vi "Machining beam pointing camera-CK(StateMachine).vi"() -> ()   [LabVIEW 2009]
uses:
  <vilib>/userDefined/High Color/IMAQdx.ctl
  <vilib>/vision/Image Controls.llb/IMAQ Image.ctl
  <vilib>/Utility/error.llb/DialogType.ctl
  <vilib>/vision/driver/IMAQdx.llb/IMAQdx Buffer Number Mode.ctl
  <vilib>/vision/driver/IMAQdx.llb/IMAQdx Camera Control Mode.ctl
  <vilib>/vision/driver/IMAQdx.llb/IMAQdx Acquisition Mode.ctl
  <vilib>/vision/NI_Vision_Development_Module.lvlib
  <vilib>/vision/driver/NI_Vision_Acquisition_Software.lvlib
  Program Files/National Instruments/LabVIEW 2009/resource/objmgr/imaqdx.rc
panel:
  out "Global Report":T1 {"Mean Value" format="%.2f"; "%" format="%.2f"; "Area (calibrated)" format="%.2f"; "Maximal Value" format="%.2f"; "Minimal Value" format="%.2f"; "Standard Variation" format="%.2f"}
  out "Intensity Graph":i16[][](graph)
  out "Buffer Number Out":u32
  out "Camera Image":T2
  in  "Tab Control":T3(tab)=enum."Aquisition"
  in  "Include DS-string\nin filename":bool
  in  "Save Images":bool
  in  "Use\nGaussian <-> Centroid":bool
  in  "Set dev Limit\nto half Spotsize":bool
  out "Laser deviation":bool
  in  "Y dev limit":dbl=20.0
  in  "X dev limit":dbl=20.0
  out "Fast Buffer Means\nGaussian Fit":T4
  in  "Fast Buffer":i32=20
  out "Fit successful":bool
  out "XY Graph":cluster{i32[], "Best Gaussian Fit":dbl[]}[](graph)
  in  "Cursor 0 and Reference":u16(ring) items=["Do nothing", "Set Cursor 0 to Reference", "Set Reference to Cursor 0", "Set Reference and Cursor 0 to actual Position"]
  in  "Pause":bool
  out "Waveform Chart":i16(graph)
  out "X centroid pos":i32
  out "Y centroid pos":i32
  out "reference X index":dbl
  out "reference Y index":dbl
  in  "Activate Autoshutter":bool
  out "Shutter Value":dbl
  in  "OK":bool
  in  "Save One Image":bool
  out "Image":T2(plugin-control)
  out "Maximal Value":sgl
  in  "X parameter bounds":T5={"amp min"=0.0, "amp max"=inf, "center min"=0.0, "center max"=1288.0, "deviation min"=0.0, "deviation max"=300.0, "offset min"=0.0, "offset max"=inf}
  in  "Y parameter bounds":T5={"amp min"=0.0, "amp max"=inf, "center min"=0.0, "center max"=964.0, "deviation min"=0.0, "deviation max"=300.0, "offset min"=0.0, "offset max"=inf}
  in  "Slow Buffer":i32=1000
  out "Failed Fits":i32
  in  "Range":cluster{"Lower value":sgl, "Upper value":sgl}={"Lower value"=128.0, "Upper value"=255.0} {"Upper value" format="%.2f"; "Lower value" format="%.2f"}
  out "Centroid":cluster{"X Centroid":sgl, "Y Centroid":sgl} {"Y Centroid" format="%.2f"; "X Centroid" format="%.2f"}
  out "Slow Buffer\n Deviations":T4
  in  "Filename":string
  in  "Autoshutter Steps":enum32{"Relative", "Absolute"}(tab)=enum."Absolute"
  in  "%":dbl=10.0
  in  "ms":dbl=100.0
  in  "Image Buffer":u32=10
  in  "Device":T6="cam1"
  in  "Autoshutter Limits":cluster{"Upper Limit":i32, "Lopwer Limit":i32}={"Upper Limit"=3500, "Lopwer Limit"=1500}
  in  "Path":path=path "C:/Temp/ImagesCK"
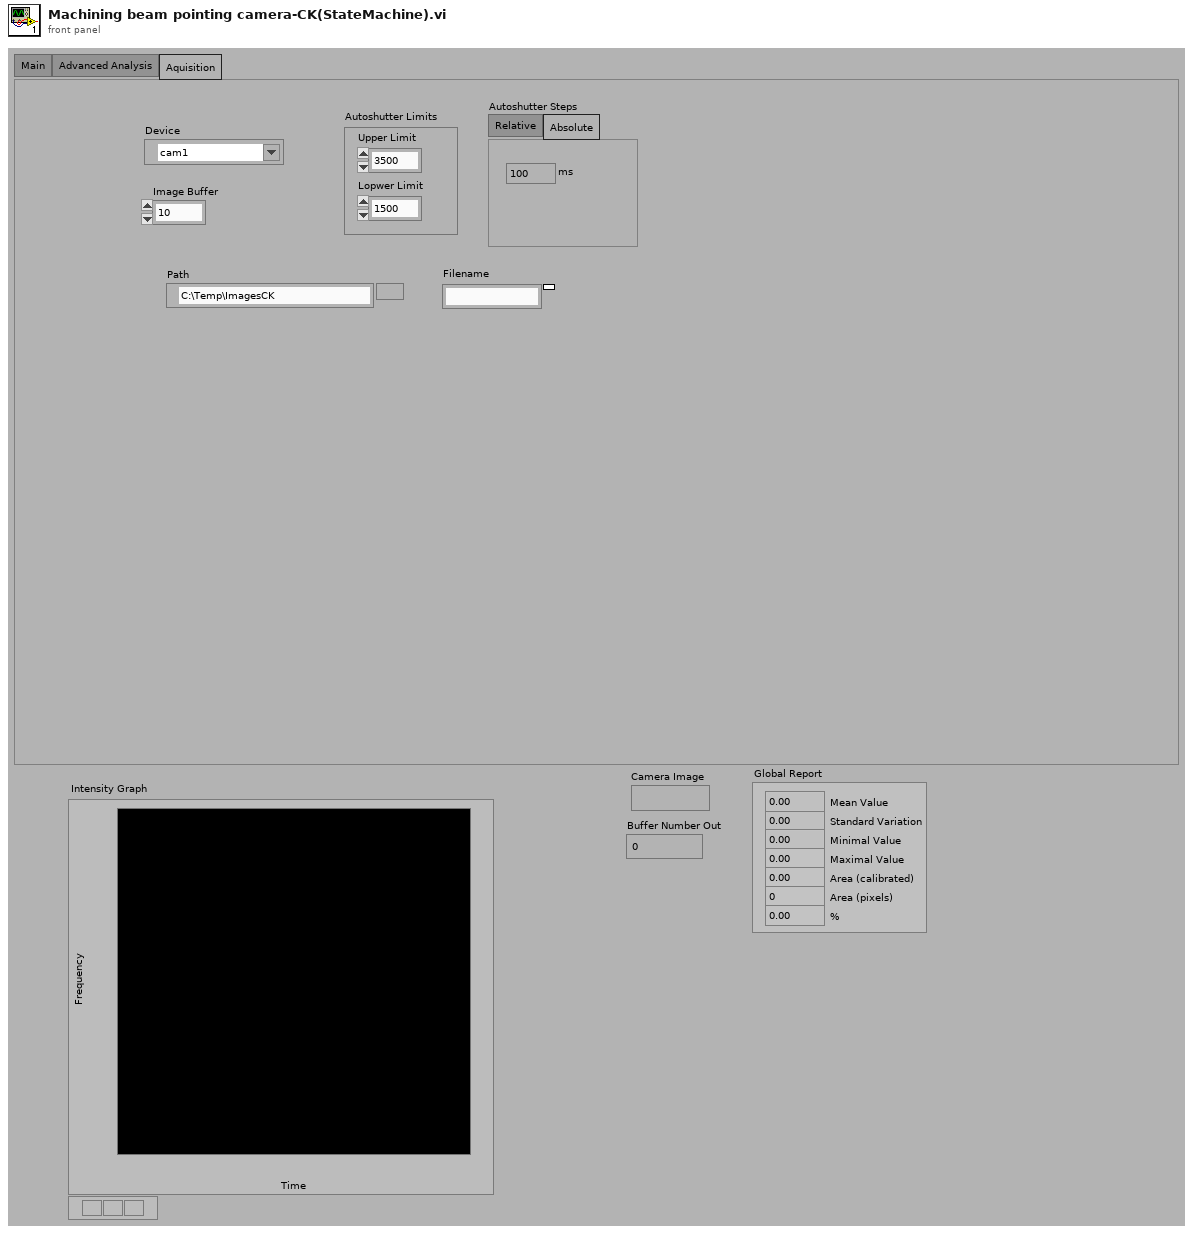
[diagram p1: front panel]
types:
  T1 = cluster{"Mean Value":sgl, "Standard Variation":sgl, "Minimal Value":sgl, "Maximal Value":sgl, "Area (calibrated)":sgl, "Area (pixels)":i32, "%":sgl}
  T2 = typedef "IMAQ Image.ctl" = refnum<image>
  T3 = enum32{"Main", "Advanced Analysis", "Aquisition"}
  T4 = cluster{"Y-AMplitude":dbl, "Y-deviation":dbl, "Y-position":dbl, "X-Amplitude":dbl, "X-deviation":dbl, "X-Position":dbl}
  T5 = cluster{"amp min":dbl, "amp max":dbl, "center min":dbl, "center max":dbl, "deviation min":dbl, "deviation max":dbl, "offset min":dbl, "offset max":dbl}
  T6 = typedef "IMAQdx.ctl" = refnum<k21>
  T7 = enum32{"invalid app kind", "Development System", "Run Time System", "Student Edition", "Embedded LabVIEW", "Evaluation", "Custom"}
  T8 = enum32{"Invalid", "Standard", "Closed", "Hidden", "Minimized", "Maximized"}
  T9 = typedef "NI_Vision_Acquisition_Software.lvlib/IMAQdx Buffer Number Mode.ctl" = enum32{"Next", "Last", "Buffer Number"}
  T10 = typedef "NI_Vision_Acquisition_Software.lvlib/IMAQdx Camera Control Mode.ctl" = enum32{"Controller", "Listener"}
  T11 = typedef "NI_Vision_Acquisition_Software.lvlib/IMAQdx Acquisition Mode.ctl" = enum32{"One Shot", "Continuous"}
  T12 = cluster{"Core":cluster{"Current VI Reference":refnum<vi>, "Close Panel on Exit?":bool}, "IMAQdx Session":T6, "Camera Image":T2, "Threshold Image":T2, "Framecount":u64, "Gaussian Result":cluster{cluster{"Y-amplitude":dbl, "Y-standard deviation":dbl, "Y-center":dbl}, cluster{"X-amplitude":dbl, "X-standard deviation":dbl, "X-center":dbl}}, "Global Report":cluster{"Mean Value":sgl, "Standard Variation":sgl, "Minimal Value":sgl, "Maximal Value":sgl, "Area (calibrated)":sgl, "Area (pixels)":i32, "%":sgl}, "Centroid":cluster{"X Centroid":sgl, "Y Centroid":sgl}, "DataBuffer":cluster{cluster{"Y-amplitude":dbl, "Y-standard deviation":dbl, "Y-center":dbl}, cluster{"X-amplitude":dbl, "X-standard deviation":dbl, "X-center":dbl}}[], "Fast Buffer Results":cluster{"Y-AMplitude":dbl, "Y-deviation":dbl, "Y-position":dbl, "X-Amplitude":dbl, "X-deviation":dbl, "X-Position":dbl}}
  T13 = typedef "DialogType.ctl" = u16
  T14 = cluster{cluster{"Y-amplitude":dbl, "Y-standard deviation":dbl, "Y-center":dbl}, cluster{"X-amplitude":dbl, "X-standard deviation":dbl, "X-center":dbl}}
  T15 = cluster{cluster{"Y-amplitude":dbl, "Y-standard deviation":dbl, "Y-center":dbl}, cluster{"X-amplitude":dbl, "X-standard deviation":dbl, "X-center":dbl}}[]
  T16 = cluster{"Current VI Reference":refnum<vi>, "Close Panel on Exit?":bool}
  T17 = cluster{"reference X index ":dbl, "reference Y index ":dbl}
  T18 = typedef "LVPointDoubleTypeDef.ctl" = cluster{"Cursor X":dbl, "Cursor Y":dbl}
  T19 = cluster{"X centroid pos":i32, "Y centroid pos":i32}
  T20 = typedef "Image Type" = u32
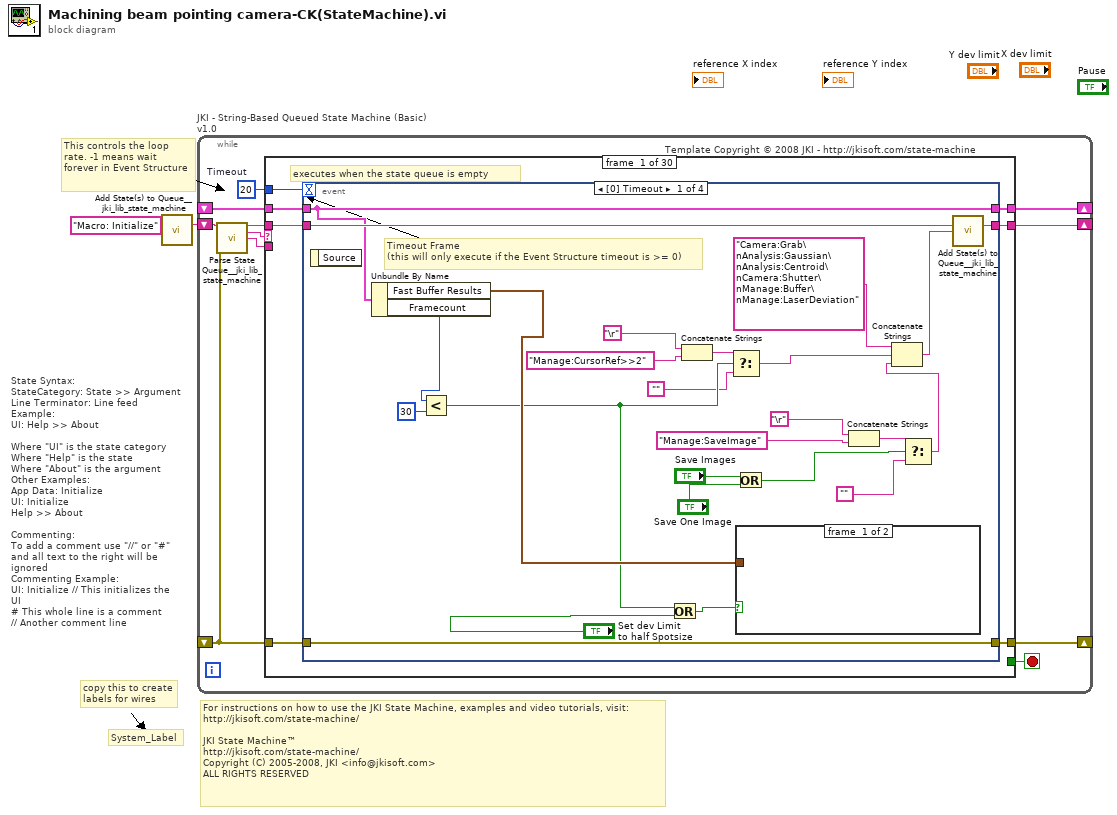
[diagram p0: block diagram]
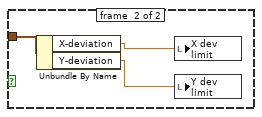
[diagram p2: hidden frame]
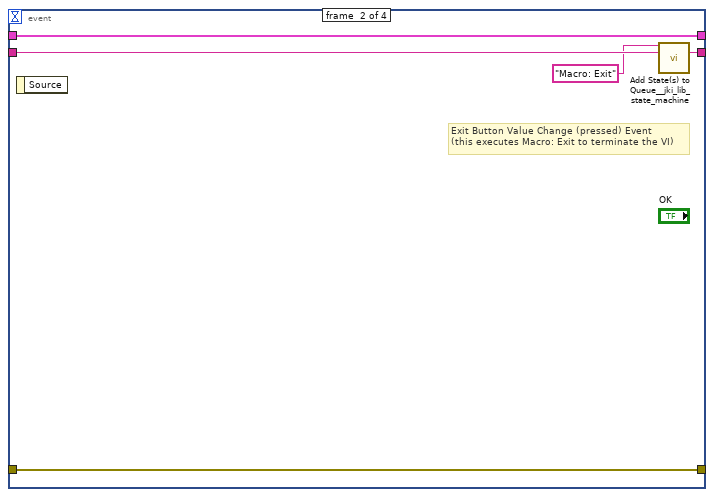
[diagram p3: hidden frame]
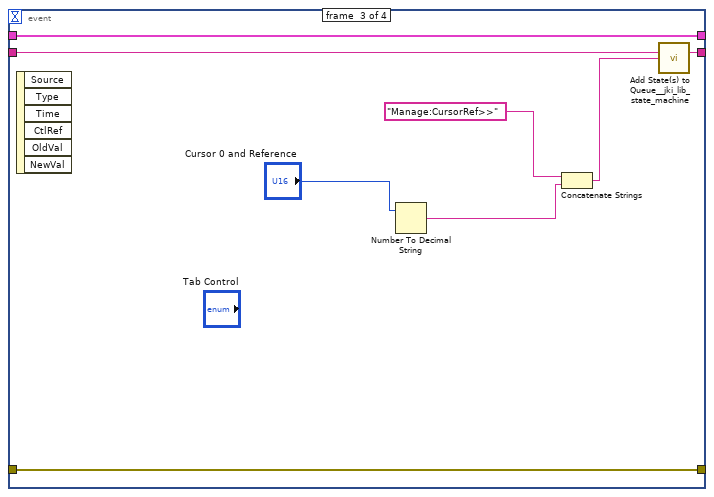
[diagram p4: hidden frame]
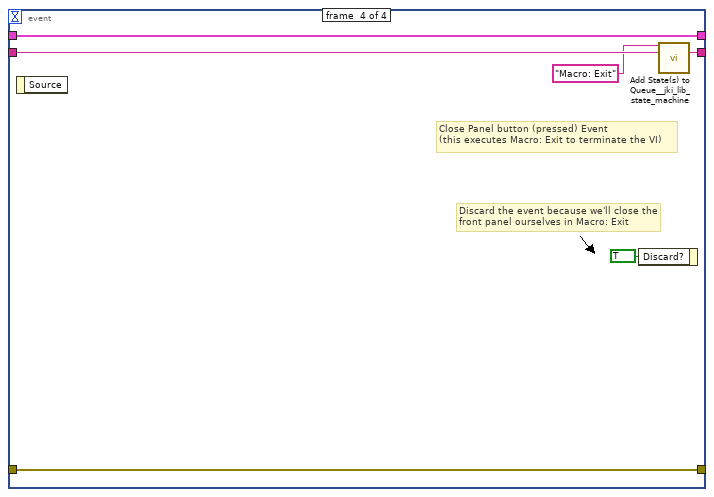
[diagram p5: hidden frame]
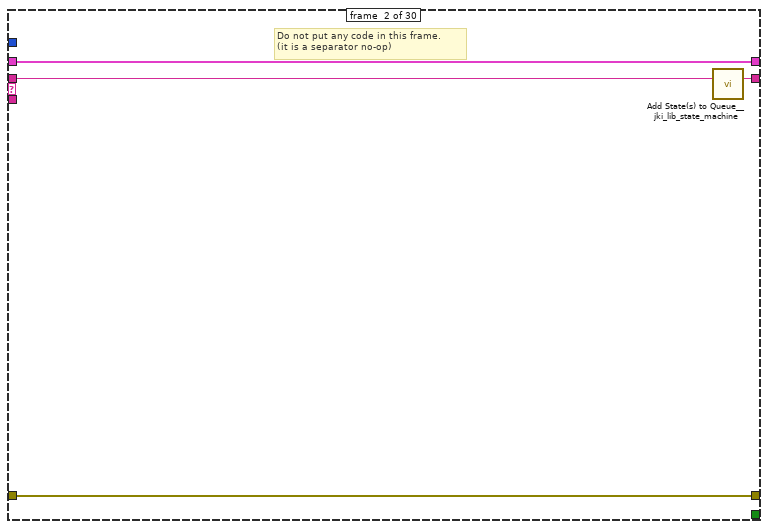
[diagram p6: hidden frame]
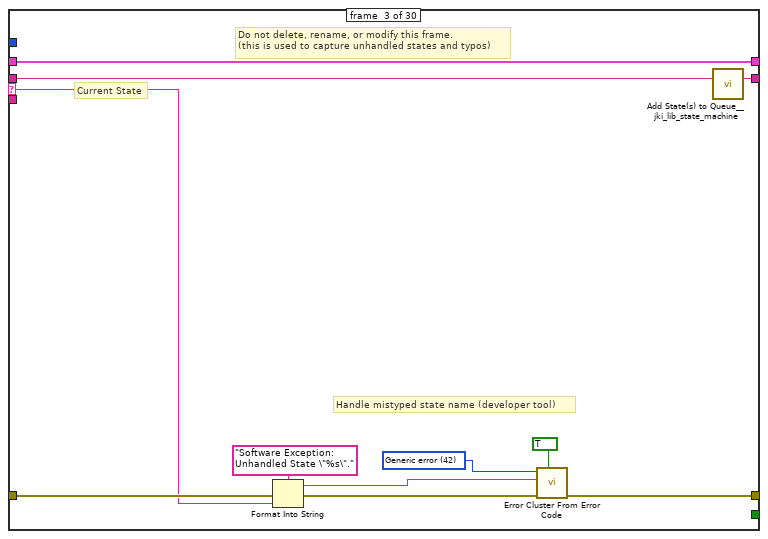
[diagram p7: hidden frame]
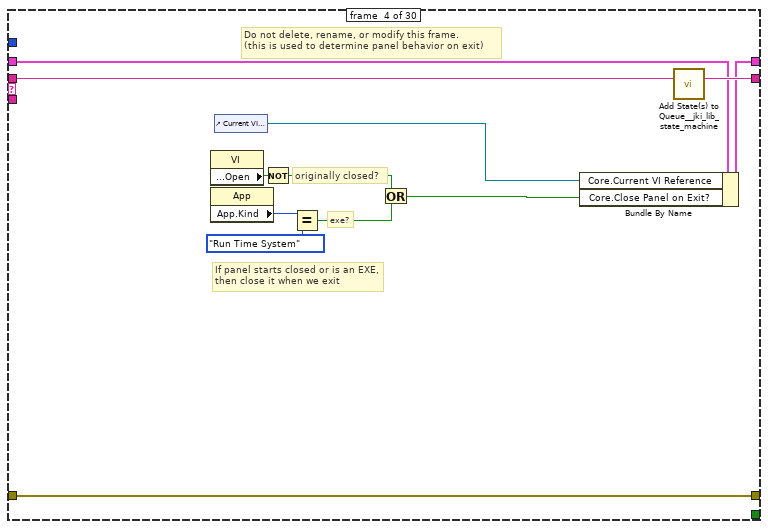
[diagram p8: hidden frame]
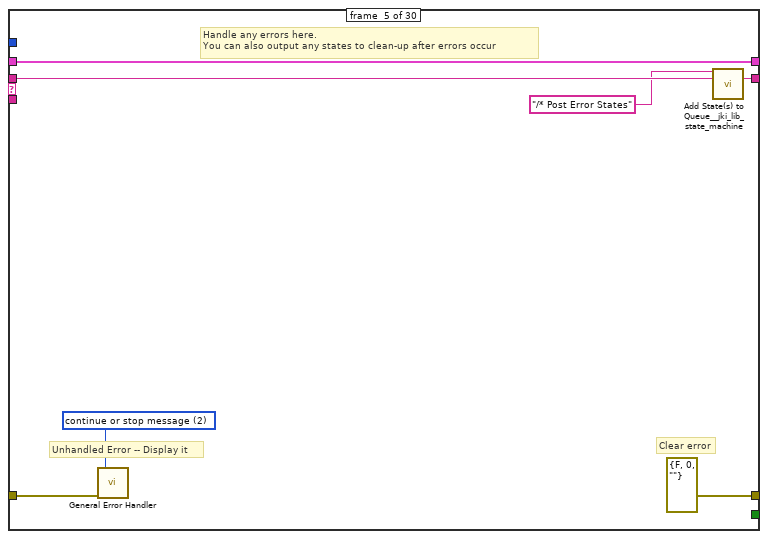
[diagram p9: hidden frame]
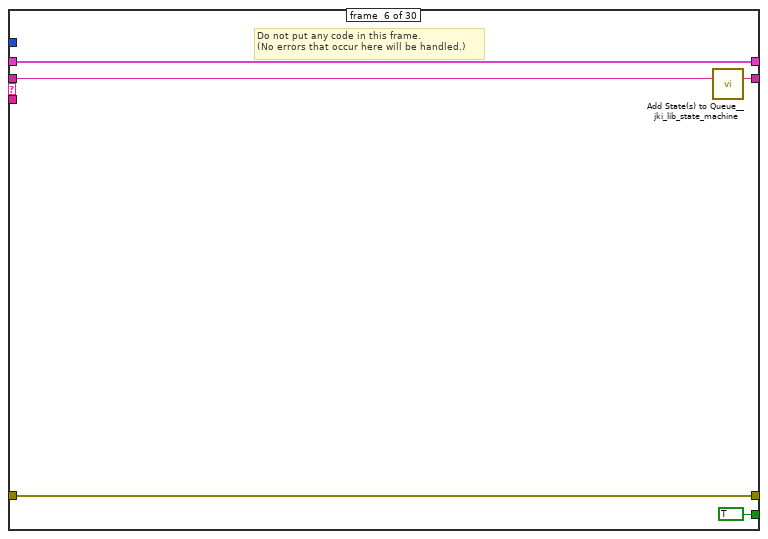
[diagram p10: hidden frame]
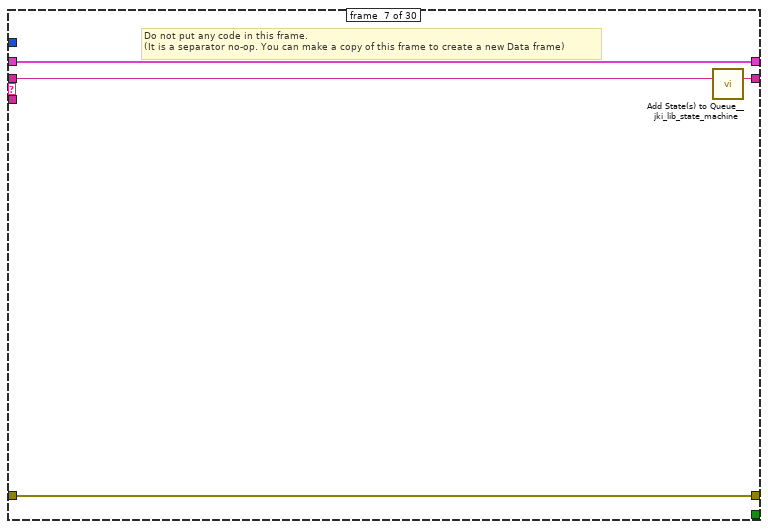
[diagram p11: hidden frame]
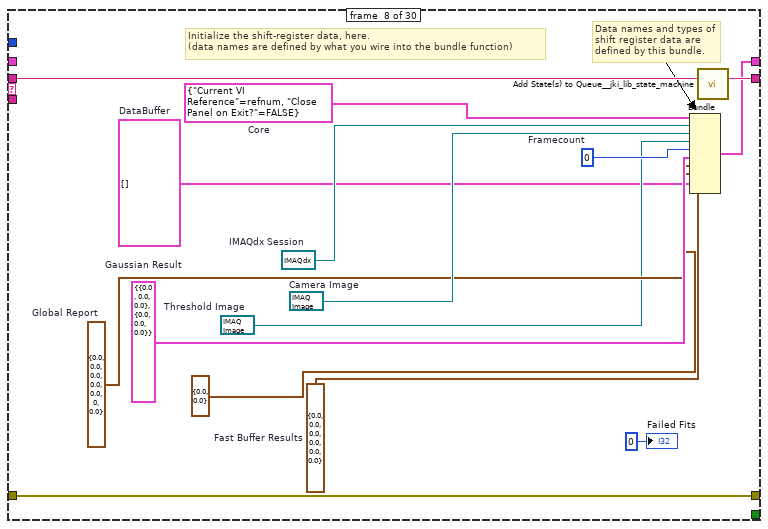
[diagram p12: hidden frame]
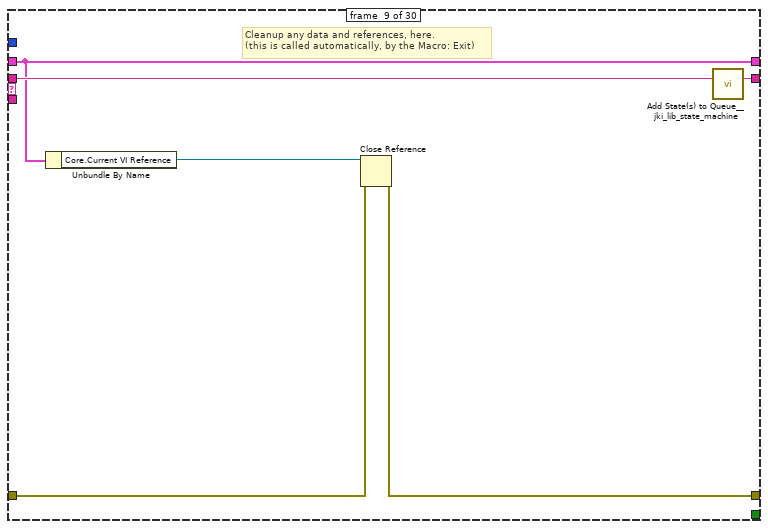
[diagram p13: hidden frame]
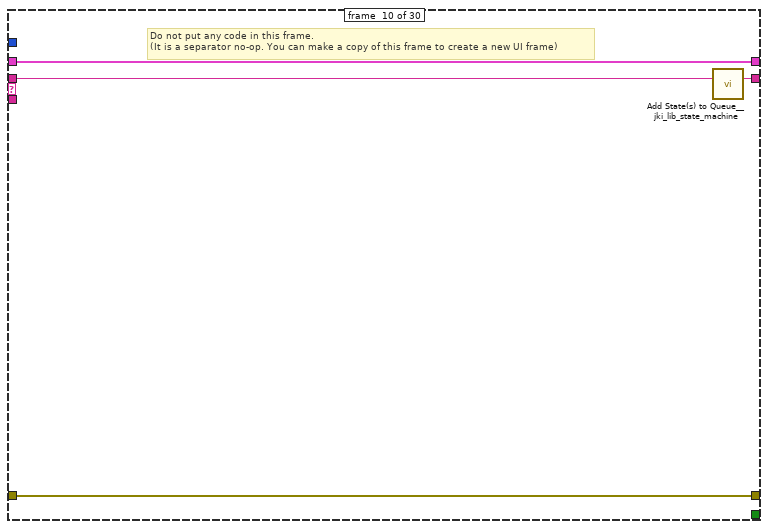
[diagram p14: hidden frame]
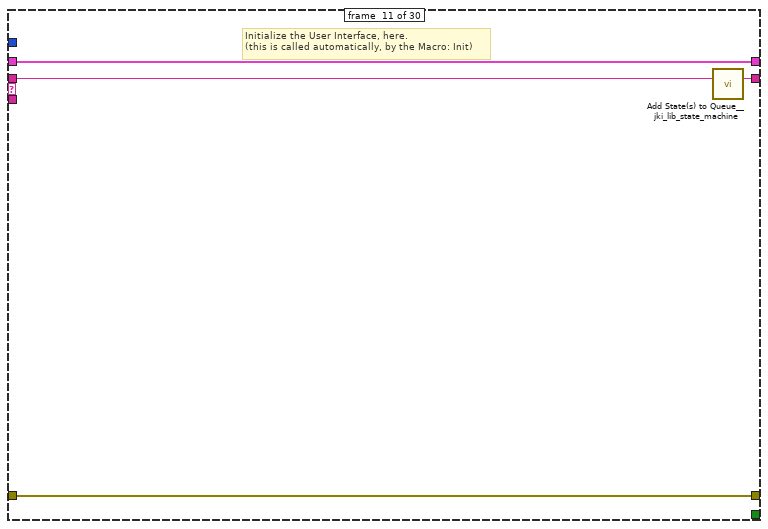
[diagram p15: hidden frame]
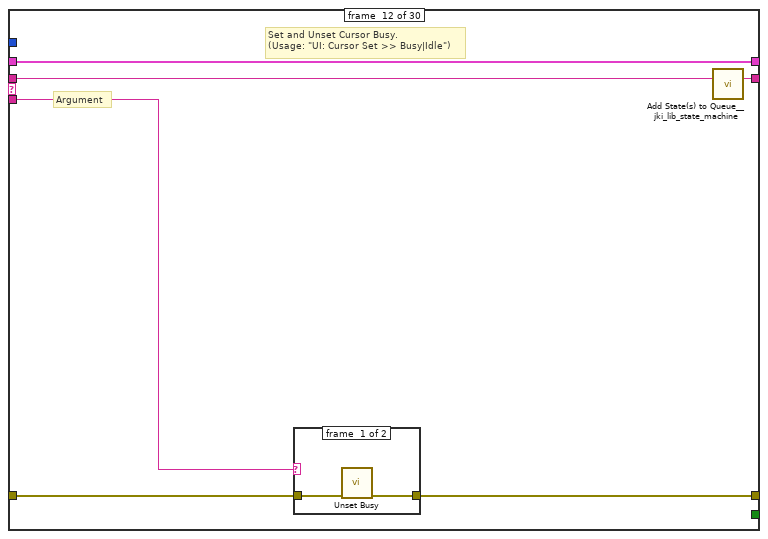
[diagram p16: hidden frame]
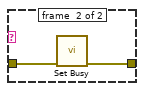
[diagram p17: hidden frame]
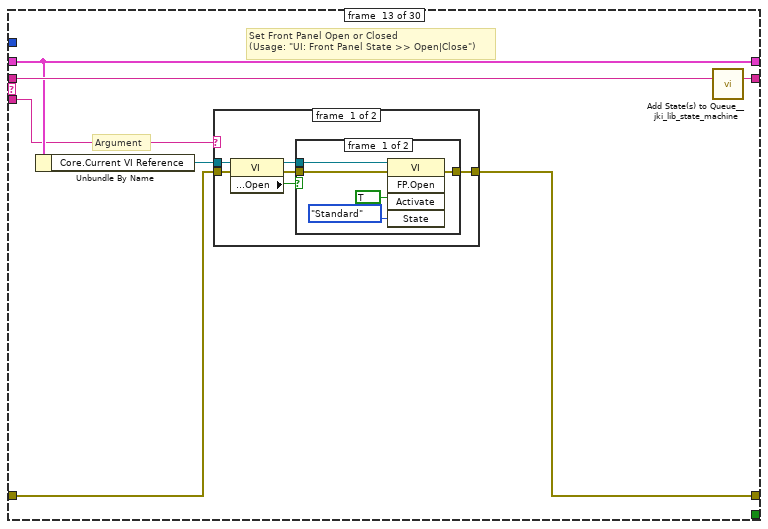
[diagram p18: hidden frame]
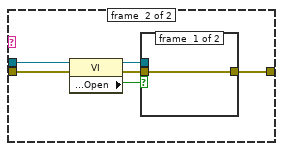
[diagram p20: hidden frame]
diagram:
  # "For instructions on how to use the JKI State Machine, examples and video tutorials, visit:\nhttp://jkisoft.com/state-machine/\n\nJKI State Machine™\nhttp://jkisoft.com/state-machine/\nCopyright (C) 2005-2008, JKI <info@jkisoft.com>\nALL RIGHTS RESERVED"
  # "State Syntax:\nStateCategory: State >> Argument\nLine Terminator: Line feed\nExample:\nUI: Help >> About\n\nWhere \"UI\" is the state category\nWhere \"Help\" is the state\nWhere \"About\" is the argument\nOther Examples:\nApp Data: Initialize\nUI: Initialize\nHelp >> About\n\nCommenting:\nTo add a comment use \"//\" or \"#\" and all text to the right will be ignored\nCommenting Example:\nUI: Initialize // This initializes the UI\n# This whole line is a comment\n// Another comment line"
  # "copy this to create labels for wires"
  # "This controls the loop rate. -1 means wait forever in Event Structure"
  # "System_Label"
  n1 = call <vilib>:"Add State(s) to Queue__jki_lib_state_machine.vi"("State(s) in (\"\")"="Macro: Initialize") -> ("States Out"=w2:string)  [unwired: 14 in]
  n2 = while "JKI - String-Based Queued State Machine (Basic) v1.0" {
    shift-right: [w6] -> _
    shift-left: _ -> [w5]
    shift-right: [w9] -> _
    shift-left: _ -> [w3]
    shift-right: [w8] -> _
    shift-left: w2 -> [w10]
    stop <- w7 stop-if-true
    w4 = 20  # Timeout
    # "Template Copyright © 2008 JKI - http://jkisoft.com/state-machine"
    n3 = call <vilib>:"Parse State Queue__jki_lib_state_machine.vi"("State Queue"=w10, "Error In (no error)"=w3) -> ("Remaining States"=w12:string, "Current State"=w13:string, "Arguments"=w11:string)  [unwired: 11 in]
    n4 = case shown="\"Analysis:Centroid\"" w13 {
      selector: w13 -> [_ _ w72 _ _ _ _ _ _ _ _ _ _ _ _ _ _ _ _ _ _ _ _ _ _ _ _ _ _ _]
      tunnel: w12 -> [w20 w71 w76 w94 w101 w106 w110 w125 w131 w135 w139 w145 w156 w182 w187 w197 w201 w236 w259 w294 w326 w330 w348 w359 w365 w369 w387 w406 w441 w452]
      tunnel: w11 -> [_ _ _ _ _ _ _ _ _ _ _ w140 w150 _ _ _ _ _ w253 _ _ _ _ _ _ _ _ _ _ _]
      tunnel: w5 -> [w18 w68 w74 w85 w98 w104 w107 _ w126 w132 w137 w143 w152 w179 w184 w194 w198 w231 w255 w282 w323 w327 w346 w356 w362 w366 w385 w404 w439 w445]
      tunnel: [w17 w69 w78 w91 errorcluster {"status"=FALSE, "code"=0, "source"=""} ("error out") w103 w108 w118 w127 w133 w136 w141 w153 w180 w185 w195 w199 w233 w256 w283 w324 w328 w333 w357 w363 w367 w375 w391 w420 w446] -> w9
      tunnel: w3 -> [w16 w69 w77 w91 w97 w103 w108 w118 w128 w133 w136 w142 w154 w180 w185 w195 w199 w222 w257 w284 w324 w328 w341 w357 w363 w367 w380 w392 w427 w444]
      tunnel: [w19 w70 w75 w93 w100 w105 w109 w124 w130 w134 w138 w144 w155 w181 w186 w196 w200 w235 w258 w293 w325 w329 w347 w358 w364 w368 w386 w405 w440 w451] -> w8
      tunnel: [_ _ _ _ _ TRUE _ _ _ _ _ _ _ _ _ _ _ _ _ _ _ _ _ _ _ _ _ _ _ _] -> w7
      tunnel: [w15 w68 w74 w92 w98 w104 w107 w123 w126 w132 w137 w143 w152 w179 w184 w194 w198 w230 w255 w282 w322 w327 w345 w355 w362 w366 w384 w403 w438 w445] -> w6
      tunnel: w4 -> [w14 _ _ _ _ _ _ _ _ _ _ _ _ _ _ _ _ _ _ _ _ _ _ _ _ _ _ _ _ _]
      frame #0 {
        # "executes when the state queue is empty"
        n5 = event shown="[0] Timeout" {
          selector: _ -> [_ _ _ _]
          dyn-events: _ -> [_ _ _ _]
          timeout: w14 -> [_ _ _ _]
          tunnel: w20 -> [w45 w53 w61 w67]
          tunnel: [w44 w52 w60 w66] -> w19
          tunnel: w18 -> [w37 w50 w58 w64]
          tunnel: [w43 w51 w59 w65] -> w17
          tunnel: w16 -> [w43 w51 w59 w65]
          tunnel: [w37 w50 w58 w64] -> w15
          event #0 {
            # "Timeout Frame\n(this will only execute if the Event Structure timeout is >= 0)"
            n6 = event-data() -> ()  [unwired: 1 in, 1 out]
            n7 = Unbundle By Name(w37) -> ("Fast Buffer Results"=w40:T4, "Framecount"=w38:u64)
            n8 = Less?(x=w38, y=u64 30) -> (x < y?=w35:bool)
            n9 = Or(x=w35, y="Set dev Limit\nto half Spotsize") -> (x .or. y?=w41:bool)
            n10 = Concatenate Strings("\r", "Manage:CursorRef>>2" ("State(s) at Back (\"\")")) -> (w31:string)
            n11 = Select(t=w31, s=w35, f="") -> (s? t:f=w30:string)
            n12 = Or(x="Save Images", y="Save One Image") -> (x .or. y?=w21:bool)
            n13 = case shown="True" w41 {
              tunnel: w40 -> [_ w46]
              frame #0 {
              }
              frame #1 {
                n14 = Unbundle By Name(w46) -> ("X-deviation"=w47:dbl, "Y-deviation"=w48:dbl)
                n15 = local write "X dev limit"(w47) -> ()
                n16 = local write "Y dev limit"(w48) -> ()
              }
            }
            n17 = Concatenate Strings("\r", "Manage:SaveImage" ("State(s) at Back (\"\")")) -> (w28:string)
            n18 = Select(t=w28, s=w21, f="") -> (s? t:f=w24:string)
            n19 = Concatenate Strings("Camera:Grab\nAnalysis:Gaussian\nAnalysis:Centroid\nCamera:Shutter\nManage:Buffer\nManage:LaserDeviation" ("State(s) at Back (\"\")"), w30, w24) -> (w29:string)
            n20 = call <vilib>:"Add State(s) to Queue__jki_lib_state_machine.vi"("State(s) in (\"\")"=w45, "State(s) at Back (\"\")"=w29) -> ("States Out"=w44:string)  [unwired: 13 in]
          }
          event #1 {
            # "Exit Button Value Change (pressed) Event\n(this executes Macro: Exit to terminate the VI)"
            n21 = event-data() -> ()  [unwired: 1 in, 1 out]
            n22 = call <vilib>:"Add State(s) to Queue__jki_lib_state_machine.vi"("State(s) in Front (\"\")"="Macro: Exit", "State(s) in (\"\")"=w53) -> ("States Out"=w52:string)  [unwired: 13 in]
          }
          event #2 {
            n23 = event-data() -> ()  [unwired: 1 in, 6 out]
            n24 = Number To Decimal String(number="Cursor 0 and Reference") -> (decimal integer string=w56:string)  [unwired: 1 in]
            n25 = Concatenate Strings("Manage:CursorRef>>" ("State(s) at Back (\"\")"), w56) -> (w54:string)
            n26 = call <vilib>:"Add State(s) to Queue__jki_lib_state_machine.vi"("State(s) in (\"\")"=w61, "State(s) at Back (\"\")"=w54) -> ("States Out"=w60:string)  [unwired: 13 in]
          }
          event #3 {
            # "Discard the event because we'll close the front panel ourselves in Macro: Exit"
            # "Close Panel button (pressed) Event\n(this executes Macro: Exit to terminate the VI)"
            n27 = event-data() -> ()  [unwired: 1 in, 1 out]
            n28 = event-data("Discard?"=TRUE) -> ()  [unwired: 1 in, 1 out]
            n29 = call <vilib>:"Add State(s) to Queue__jki_lib_state_machine.vi"("State(s) in Front (\"\")"="Macro: Exit", "State(s) in (\"\")"=w67) -> ("States Out"=w66:string)  [unwired: 13 in]
          }
        }
      }
      frame #1 {
        # "Do not put any code in this frame.\n(it is a separator no-op)"
        n30 = call <vilib>:"Add State(s) to Queue__jki_lib_state_machine.vi"("State(s) in (\"\")"=w71) -> ("States Out"=w70:string)  [unwired: 14 in]
      }
      frame #2 {
        w81 = 42 items=["No error", "Argument error", "Memory is full", "Out of zone", "End of file", "File already open", "Generic file I/O error", "File not found", "File permission error", "Disk is full", "Duplicate path", "Too many files open", "System feature not enabled", "Resource file not found", "Cannot add resource", "Resource not found", "Image not found", "Image memory error", "Pen does not exist", "Config type invalid", "Config token not found", "Config parse error", "Config memory error", "Bad external code format", "Bad external code offset", "External code not present", "Null window", "Destroy window error", "Null menu", "Print aborted", "Bad print record", "Print driver error", "Windows error during printing", "Memory error during printing", "Print dialog error", "Generic print error", "Invalid device refnum", "Device not found", "Device parameter error", "Device unit error", "Cannot open device", "Device call aborted", "Generic error", "Cancelled by user", "Object ID too low", "Object ID too high", "Object not in heap", "Unknown heap", "Unknown object (invalid DefProc)", "Unknown object (DefProc not in table)", "Message out of range", "Invalid (null) method", "Unknown message", "Manager call not supported", "Bad address", "Network operation in progress", "Network operation timed out", "Connection is busy", "Network attribute not supported", "Network error", "Address in use", "System out of memory", "Connection aborted", "Connection refused", "Not connected", "Already connected", "Connection closed", "Initialization error (interapplication manager)", "Bad occurrence", "Wait on unbound occurrence handler", "Occurrence queue overflow", "Datalog type conflict", "Unused", "Unrecognized type (interapplication manager)", "Memory corrupt", "Failed to make temporary DLL", "Old CIN version", "Drag socket not found", "Failed to load drop-object", "Failed to register OLE object", "Failed to release OLE object", "Format specifier type mismatch", "Unknown format specifier", "Too few format specifiers", "Too many format specifiers", "Scan failed", "Newer CIN version", "Error converting to variant", "Runtime menu error", "Password tampered", "Variant attribute not found", "Incompatible variant data type", "Event data is not available", "Event Store is not present", "Occurrence is not found", "Event Queue is not created", "Event info is not available", "Refnum passed is NULL", "Error retrieving Class GUID", "Error retrieving CoClass GUID", "Error retrieving TypeLib GUID.", "Bad built application magic bytes.", "Specific driver is different from the specific driver associated with the Logical Name.", "There is no session opened to the class driver.", "Max Error", "MAX - Error with config objects", "MAX - Error loading configuration", "MAX - Group not supported"]
        # "Current State"
        # "Do not delete, rename, or modify this frame.\n(this is used to capture unhandled states and typos)"
        # "Handle mistyped state name (developer tool)"
        n31 = Format Into String(format string="Software Exception: Unhandled State \"%s\"." ("message"), error in=w77, w72) -> (resulting string=w80:string, error out=w79:errorcluster)  [unwired: 1 in]
        n32 = call <vilib>:"Error Cluster From Error Code.vi"("show call chain? (False)"=TRUE, "error in (no error)"=w79, "error message (\"\")"=w80, "error code (0)"=w81) -> ("error out"=w78:errorcluster)  [unwired: 5 in]
        n33 = call <vilib>:"Add State(s) to Queue__jki_lib_state_machine.vi"("State(s) in (\"\")"=w76) -> ("States Out"=w75:string)  [unwired: 14 in]
      }
      frame #3 {
        # "Do not delete, rename, or modify this frame.\n(this is used to determine panel behavior on exit)"
        # "originally closed?"
        # "exe?"
        # "If panel starts closed or is an EXE, then close it when we exit"
        n34 = property class="VI"() -> ("Front Panel.Open"=w90:bool)  [unwired: 2 in, 2 out]
        n35 = property class="App"() -> ("App.Kind"=w89:T7)  [unwired: 2 in, 2 out]
        n36 = control-ref of="Current VI Reference"() -> (w83:refnum<vi>)
        n37 = Not(x=w90) -> (.not. x?=w87:bool)
        n38 = Equal?(x=w89, y=T7."Run Time System" ("Application:Kind")) -> (x = y?=w86:bool)
        n39 = Or(x=w87, y=w86) -> (x .or. y?=w84:bool)
        n40 = Bundle By Name(cluster=w85, "Core.Current VI Reference"=w83, "Core.Close Panel on Exit?"=w84) -> (w92:T12)
        n41 = call <vilib>:"Add State(s) to Queue__jki_lib_state_machine.vi"("State(s) in (\"\")"=w94) -> ("States Out"=w93:string)  [unwired: 14 in]
      }
      frame #4 {
        w95 = T13 2 items=["no dialog", "OK message", "continue or stop message", "OK message + warnings", "continue/stop + warnings"] ("type of dialog (OK msg:1)")
        # "Unhandled Error -- Display it"
        # "Handle any errors here.\nYou can also output any states to clean-up after errors occur"
        # "Clear error"
        n42 = call <vilib>:"General Error Handler.vi"("type of dialog (OK msg:1)"=w95, "error in (no error)"=w97) -> ()  [unwired: 9 in, 5 out]
        n43 = call <vilib>:"Add State(s) to Queue__jki_lib_state_machine.vi"("State(s) in Front (\"\")"="/* Post Error States", "State(s) in (\"\")"=w101) -> ("States Out"=w100:string)  [unwired: 13 in]
      }
      frame #5 {
        # "Do not put any code in this frame.\n(No errors that occur here will be handled.)"
        n44 = call <vilib>:"Add State(s) to Queue__jki_lib_state_machine.vi"("State(s) in (\"\")"=w106) -> ("States Out"=w105:string)  [unwired: 14 in]
      }
      frame #6 {
        # "Do not put any code in this frame.\n(It is a separator no-op. You can make a copy of this frame to create a new Data frame)"
        n45 = call <vilib>:"Add State(s) to Queue__jki_lib_state_machine.vi"("State(s) in (\"\")"=w110) -> ("States Out"=w109:string)  [unwired: 14 in]
      }
      frame #7 {
        w112 = T4 {"Y-AMplitude"=0.0, "Y-deviation"=0.0, "Y-position"=0.0, "X-Amplitude"=0.0, "X-deviation"=0.0, "X-Position"=0.0}  # Fast Buffer Results
        w114 = T2 refnum  # Threshold Image
        w116 = T1 {"Mean Value"=0.0, "Standard Variation"=0.0, "Minimal Value"=0.0, "Maximal Value"=0.0, "Area (calibrated)"=0.0, "Area (pixels)"=0, "%"=0.0}  # Global Report
        w117 = T14 {{"Y-amplitude"=0.0, "Y-standard deviation"=0.0, "Y-center"=0.0}, {"X-amplitude"=0.0, "X-standard deviation"=0.0, "X-center"=0.0}}  # Gaussian Result
        w119 = T2 refnum  # Camera Image
        w120 = T6 refnum  # IMAQdx Session
        w121 = u64 0  # Framecount
        w113 = T15 []  # DataBuffer
        w122 = T16 {"Current VI Reference"=refnum, "Close Panel on Exit?"=FALSE}  # Core
        # "Data names and types of shift register data are defined by this bundle."
        # "Initialize the shift-register data, here.\n(data names are defined by what you wire into the bundle function)"
        n46 = Bundle("Core"=w122, "IMAQdx Session"=w120, "Camera Image"=w119, "Threshold Image"=w114, "Framecount"=w121, "Gaussian Result"=w117, "Global Report"=w116, "Centroid"=cluster{"X Centroid":sgl, "Y Centroid":sgl} {"X Centroid"=0.0, "Y Centroid"=0.0}, "DataBuffer"=w113, "Fast Buffer Results"=w112) -> (w123:T12)  [unwired: 1 in]
        n47 = call <vilib>:"Add State(s) to Queue__jki_lib_state_machine.vi"("State(s) in (\"\")"=w125) -> ("States Out"=w124:string)  [unwired: 14 in]
        "Failed Fits" <- 0 ("Failed Fits")
      }
      frame #8 {
        # "Cleanup any data and references, here.\n(this is called automatically, by the Macro: Exit)"
        n48 = Unbundle By Name(w126) -> ("Core.Current VI Reference"=w129:refnum<vi>)
        n49 = Close Reference(reference=w129, error in (no error)=w128) -> (error out=w127:errorcluster)
        n50 = call <vilib>:"Add State(s) to Queue__jki_lib_state_machine.vi"("State(s) in (\"\")"=w131) -> ("States Out"=w130:string)  [unwired: 14 in]
      }
      frame #9 {
        # "Do not put any code in this frame.\n(It is a separator no-op. You can make a copy of this frame to create a new UI frame)"
        n51 = call <vilib>:"Add State(s) to Queue__jki_lib_state_machine.vi"("State(s) in (\"\")"=w135) -> ("States Out"=w134:string)  [unwired: 14 in]
      }
      frame #10 {
        # "Initialize the User Interface, here.\n(this is called automatically, by the Macro: Init)"
        n52 = call <vilib>:"Add State(s) to Queue__jki_lib_state_machine.vi"("State(s) in (\"\")"=w139) -> ("States Out"=w138:string)  [unwired: 14 in]
      }
      frame #11 {
        # "Argument"
        # "Set and Unset Cursor Busy.\n(Usage: \"UI: Cursor Set >> Busy|Idle\")"
        n53 = case shown="\"Idle\", Default" w140 {
          tunnel: w142 -> [w147 w149]
          tunnel: [w146 w148] -> w141
          frame #0 {
            n54 = call <vilib>:"Unset Busy.vi"("error in (no error)"=w147) -> ("error out"=w146:errorcluster)  [unwired: 10 in]
          }
          frame #1 {
            n55 = call <vilib>:"Set Busy.vi"("error in (no error)"=w149) -> ("error out"=w148:errorcluster)  [unwired: 9 in, 1 out]
          }
        }
        n56 = call <vilib>:"Add State(s) to Queue__jki_lib_state_machine.vi"("State(s) in (\"\")"=w145) -> ("States Out"=w144:string)  [unwired: 14 in]
      }
      frame #12 {
        # "Argument"
        # "Set Front Panel Open or Closed\n(Usage: \"UI: Front Panel State >> Open|Close\")"
        n57 = Unbundle By Name(w152) -> ("Core.Current VI Reference"=w151:refnum<vi>)
        n58 = case shown="\"Open\", Default" w150 {
          tunnel: w154 -> [w160 w173]
          tunnel: [w162 w174] -> w153
          tunnel: w151 -> [w161 w171]
          frame #0 {
            n59 = property class="VI"(reference=w161, error in=w160) -> (reference out=w158:refnum<vi>, error out=w159:errorcluster, "Front Panel.Open"=w157:bool)
            n60 = case shown="False" w157 {
              tunnel: [w165 w168] -> w162
              tunnel: w159 -> [w164 w168]
              tunnel: w158 -> [w163 _]
              frame #0 {
                n61 = invoke class="VI" method="FP.Open"(reference=w163, error in=w164, "Activate"=TRUE, "State"=T8."Standard") -> (error out=w165:errorcluster)  [unwired: 1 in, 4 out]
              }
              frame #1 {
              }
            }
          }
          frame #1 {
            n62 = property class="VI"(reference=w171, error in=w173) -> (reference out=w170:refnum<vi>, error out=w172:errorcluster, "Front Panel.Open"=w169:bool)
            n63 = case shown="True" w169 {
              tunnel: [w175 w178] -> w174
              tunnel: w172 -> [w175 w177]
              tunnel: w170 -> [_ w176]
              frame #0 {
              }
              frame #1 {
                n64 = invoke class="VI" method="FP.Close"(reference=w176, error in=w177) -> (error out=w178:errorcluster)  [unwired: 1 in, 2 out]
              }
            }
          }
        }
        n65 = call <vilib>:"Add State(s) to Queue__jki_lib_state_machine.vi"("State(s) in (\"\")"=w156) -> ("States Out"=w155:string)  [unwired: 14 in]
      }
      frame #13 {
        # "Do not put any code in this frame.\n(It is a separator no-op. You can make a copy of this frame to create a new Macro frame)"
        n66 = call <vilib>:"Add State(s) to Queue__jki_lib_state_machine.vi"("State(s) in (\"\")"=w182) -> ("States Out"=w181:string)  [unwired: 14 in]
      }
      frame #14 {
        w183 = "Data: Initialize\nInitialize Core Data\nUI: Initialize\nUI: Front Panel State >> Open\nCamera:Init"  # Data: Initialize Initialize Core Data UI: Initialize UI: Front Panel State >> Open Camera:Init
        # "Initialization Macro\n(This is called once, when the VI starts)"
        n67 = call <vilib>:"Add State(s) to Queue__jki_lib_state_machine.vi"("State(s) in Front (\"\")"=w183, "State(s) in (\"\")"=w187) -> ("States Out"=w186:string)  [unwired: 13 in]
      }
      frame #15 {
        # "Exit Macro\n(This is called once, when the VI exits)"
        n68 = Unbundle By Name(w194) -> ("Core.Close Panel on Exit?"=w193:bool)
        n69 = Select(t="UI: Front Panel State >> Close", s=w193, f="") -> (s? t:f=w190:string)
        n70 = call <vilib>:"Add State(s) to Queue__jki_lib_state_machine.vi"("State(s) in (\"\")"=w190, "State(s) at Back (\"\")"="Camera:Close\nData: Cleanup\nExit") -> ("States Out"=w188:string)  [unwired: 13 in]
        n71 = call <vilib>:"Add State(s) to Queue__jki_lib_state_machine.vi"("State(s) in Front (\"\")"=w188, "State(s) in (\"\")"=w197) -> ("States Out"=w196:string)  [unwired: 13 in]
      }
      frame #16 {
        # "Template Separator\n(You can make a copy of, or modify, this frame)"
        n72 = call <vilib>:"Add State(s) to Queue__jki_lib_state_machine.vi"("State(s) in (\"\")"=w201) -> ("States Out"=w200:string)  [unwired: 14 in]
      }
      frame #17 {
        # "Template Separator\n(You can make a copy of, or modify, this frame)"
        n73 = Get Date/Time In Seconds() -> (seconds since 1Jan1904=w229:timestamp)
        n74 = Unbundle By Name(w231) -> ("Camera Image"=w234:T2, "Framecount"=w226:u64)
        n75 = Get Date/Time String(seconds (now)=w229, want seconds? (F)=TRUE) -> (date string=w228:string, time string=w227:string)  [unwired: 1 in]
        n76 = Number To Decimal String(number=w226) -> (decimal integer string=w225:string)  [unwired: 1 in]
        n77 = case shown="True" "Include DS-string\nin filename" {
          tunnel: ["" w238] -> w203
          frame #0 {
          }
          frame #1 {
            w243 = TRUE ("replace all? (F)")
            n78 = Search and Replace String(replace all?=w243, case sensitive?=w243, input string="Filename", search string="[<>:\"/|?*\\\\]", replace string="_" ("replace string (\"\")")) -> (result string=w239:string)  [unwired: 3 in, 3 out]
            n79 = Concatenate Strings("_" ("string"), w239) -> (w238:string)
          }
        }
        n80 = Concatenate Strings(w228, w227, w225, w203, ".bmp" ("string")) -> (w213:string)
        n81 = call <vilib>:"Check if File or Folder Exists.vi"("error in (no error)"=w222, "path"="Path") -> ("error out"=w221:errorcluster, "file or folder exists?"=w218:bool)  [unwired: 7 in, 1 out]
        n82 = Search and Replace String(replace all?=TRUE ("replace all? (F)"), input string=w213, search string="/", replace string="_" ("replace string (\"\")")) -> (result string=w210:string)  [unwired: 4 in, 3 out]
        n83 = Search and Replace String(replace all?=TRUE ("replace all? (F)"), input string=w210, search string=":", replace string="_" ("replace string (\"\")")) -> (result string=w204:string)  [unwired: 4 in, 3 out]
        n84 = Build Path(base path="Path", name or relative path=w204) -> (appended path=w223:path)
        n85 = call <vilib>:"Check if File or Folder Exists.vi"("error in (no error)"=w221, "path"=w223) -> ("error out"=w220:errorcluster, "file or folder exists?"=w217:bool, "dup path"=w219:path)  [unwired: 7 in]
        n86 = Not(x=w217) -> (.not. x?=w216:bool)
        n87 = And(x=w216, y=w218) -> (x .and. y?=w215:bool)
        n88 = case shown="True" w215 {
          tunnel: w234 -> [w246 w252]
          tunnel: [w247 w251] -> w233
          tunnel: [w246 w250] -> w232
          tunnel: w220 -> [w247 w249]
          tunnel: w219 -> [_ w248]
          frame #0 {
            n89 = call "Display Message to User"() -> ()  [unwired: 10 in, 2 out]
            n90 = property on="Save Images" class="Bool (strict)"("Value"=FALSE ("Save Images")) -> ()  [unwired: 2 in, 2 out]
          }
          frame #1 {
            n91 = call-poly "IMAQ Write File 2"("error in (no error)"=w249, "File Path"=w248, "Image"=w252) -> ("error out"=w251:errorcluster, "Image Out (duplicate)"=w250:T2)  [unwired: 7 in]
          }
        }
        n92 = Bundle By Name(cluster=w231, "Camera Image"=w232) -> (w230:T12)
        n93 = call <vilib>:"Add State(s) to Queue__jki_lib_state_machine.vi"("State(s) in (\"\")"=w236) -> ("States Out"=w235:string)  [unwired: 14 in]
      }
      frame #18 {
        n94 = Decimal String To Number(string=w253) -> (number=w254:i32)  [unwired: 2 in, 1 out]
        n95 = case "Cursor & Reference" shown="1" w254 {
          tunnel: w257 -> [w260 w262 w269 w276]
          tunnel: [w260 w261 w268 w275] -> w256
          frame #0 {
          }
          frame #1 {
            n96 = local read "reference X index"() -> (w263:dbl)
            n97 = local read "reference Y index"() -> (w264:dbl)
            n98 = property on="Intensity Graph" class="IntGraph (strict)"(error in=w262, "Active Cursor"=u32 0) -> (error out=w265:errorcluster)  [unwired: 1 in, 1 out]
            n99 = Bundle("reference X index"=w263, "reference Y index"=w264) -> (w266:T17)  [unwired: 1 out]
            n100 = property on="Intensity Graph" class="IntGraph (strict)"(error in=w265, "Cursor.Cursor Position"=w266) -> (error out=w261:errorcluster)  [unwired: 1 in, 1 out]
          }
          frame #2 {
            n101 = property on="Intensity Graph" class="IntGraph (strict)"(error in=w269, "Active Cursor"=u32 0) -> (error out=w273:errorcluster)  [unwired: 1 in, 1 out]
            n102 = property on="Intensity Graph" class="IntGraph (strict)"(error in=w273) -> (error out=w268:errorcluster, "Cursor.Cursor Position"=w272:T18)  [unwired: 1 in, 1 out]
            n103 = Unbundle By Name(w272) -> ("Cursor X"=w271:dbl, "Cursor Y"=w270:dbl)
            n104 = local write "reference X index"(w271) -> ()
            n105 = local write "reference Y index"(w270) -> ()
          }
          frame #3 {
            n106 = local read "Y centroid pos"() -> (w277:i32)
            n107 = local read "X centroid pos"() -> (w279:i32)
            n108 = local write "reference Y index"(w277) -> ()
            n109 = property on="Intensity Graph" class="IntGraph (strict)"(error in=w276, "Active Cursor"=u32 0) -> (error out=w280:errorcluster)  [unwired: 1 in, 1 out]
            n110 = local write "reference X index"(w279) -> ()
            n111 = Bundle("X centroid pos"=w279, "Y centroid pos"=w277) -> (w278:T19)  [unwired: 1 out]
            n112 = property on="Intensity Graph" class="IntGraph (strict)"(error in=w280, "Cursor.Cursor Position"=w278) -> (error out=w275:errorcluster)  [unwired: 1 in, 1 out]
          }
        }
        n113 = call <vilib>:"Add State(s) to Queue__jki_lib_state_machine.vi"("State(s) in (\"\")"=w259) -> ("States Out"=w258:string)  [unwired: 14 in]
      }
      frame #19 {
        n114 = Unbundle By Name(w282) -> ("Fast Buffer Results"=w291:T4, "Centroid"=w290:cluster{"X Centroid":sgl, "Y Centroid":sgl})
        n115 = case shown="False" "Use\nGaussian <-> Centroid" {
          tunnel: w290 -> [_ w300]
          tunnel: w291 -> [w295 _]
          tunnel: [w297 w299] -> w286
          tunnel: [w296 w298] -> w285
          frame #0 {
            n116 = Unbundle By Name(w295) -> ("X-Position"=w297:dbl, "Y-position"=w296:dbl)
          }
          frame #1 {
            n117 = Unbundle(w300) -> ("X Centroid"=w299:sgl, "Y Centroid"=w298:sgl)
          }
        }
        n118 = flat-sequence {
          tunnel: w286 -> [w313]
          tunnel: w285 -> [w312]
          frame #0 {
            # "Check if Inbound"
            n119 = local read "reference X index"() -> (w305:dbl)
            n120 = local read "reference Y index"() -> (w304:dbl)
            n121 = local read "Y dev limit"() -> (w302:dbl)
            n122 = Subtract(x=w313, y=w305) -> (x-y=w311:dbl)
            n123 = Subtract(x=w312, y=w304) -> (x-y=w310:dbl)
            n124 = local read "X dev limit"() -> (w301:dbl)
            n125 = Absolute Value(x=w311) -> (abs(x)=w309:dbl)
            n126 = Absolute Value(x=w310) -> (abs(x)=w303:dbl)
            n127 = Greater Or Equal?(x=w309, y=w301) -> (x >= y?=w308:bool)
            n128 = Greater Or Equal?(x=w303, y=w302) -> (x >= y?=w307:bool)
            n129 = Or(x=w308, y=w307) -> (x .or. y?=→"Laser deviation":bool)
          }
        }
        n130 = Bundle("X-Position"=w286, "Y-position"=w285) -> (w288:cluster{"X-Position":dbl, "Y-position":dbl})  [unwired: 1 out]
        n131 = property on="Intensity Graph" class="IntGraph (strict)"(error in=w284, "Active Cursor"=u32 1) -> (error out=w289:errorcluster)  [unwired: 1 in, 1 out]
        n132 = property on="Intensity Graph" class="IntGraph (strict)"(error in=w289, "Cursor.Cursor Position"=w288) -> (error out=w283:errorcluster)  [unwired: 1 in, 1 out]
        n133 = call <vilib>:"Add State(s) to Queue__jki_lib_state_machine.vi"("State(s) in (\"\")"=w294) -> ("States Out"=w293:string)  [unwired: 14 in]
      }
      frame #20 {
        # "Buffer Management"
        n134 = Unbundle By Name(w323) -> ("DataBuffer"=w318:T15, "Framecount"=w317:u64, "Gaussian Result"=w315:T14)
        n135 = call "manage Buffer.vi"("Cluster"=w315, "Buffer in"=w318, "Main Index"=w317, "Analysis Buffersize"="Slow Buffer") -> ("Buffer out"=w316:T15)  [unwired: 2 in]
        n136 = call "Average_Buffer.vi"("N_Elements"="Slow Buffer", "Index"=w317, "Buffersize"="Slow Buffer", "Buffer in"=w316) -> ("output devs"=→"Slow Buffer\n Deviations":T4)  [unwired: 1 in, 1 out]
        n137 = call "Average_Buffer.vi"("N_Elements"="Fast Buffer", "Index"=w317, "Buffersize"="Slow Buffer", "Buffer in"=w316) -> ("output means"=w314:T4)  [unwired: 1 in, 1 out]
        "Fast Buffer Means\nGaussian Fit" <- w314
        n138 = Bundle By Name(cluster=w323, "DataBuffer"=w316, "Fast Buffer Results"=w314) -> (w322:T12)
        n139 = call <vilib>:"Add State(s) to Queue__jki_lib_state_machine.vi"("State(s) in (\"\")"=w326) -> ("States Out"=w325:string)  [unwired: 14 in]
      }
      frame #21 {
        # "Your code here.\n(You can make a copy of, or modify, this frame)"
        n140 = call <vilib>:"Add State(s) to Queue__jki_lib_state_machine.vi"("State(s) in (\"\")"=w330) -> ("States Out"=w329:string)  [unwired: 14 in]
      }
      frame #22 {
        n141 = Unbundle By Name(w346) -> ("Camera Image"=w335:T2, "Threshold Image"=w337:T2)
        n142 = call "IMAQ Quantify"("error in (no error)"=w341, "Image"=w335) -> ("Global Report"=w342:T1)  [unwired: 1 in, 2 out]
        n143 = call "IMAQ Threshold"("Range"="Range", "Image Dst"=w337, "Image Src"=w335) -> ("error out"=w344:errorcluster, "Image Dst Out"=w336:T2)  [unwired: 3 in, 4 out]
        n144 = call "IMAQ Centroid"("error in (no error)"=w344, "Image"=w336) -> ("error out"=w334:errorcluster, "Centroid"=w340:cluster{"X Centroid":sgl, "Y Centroid":sgl})  [unwired: 1 in, 1 out]
        "Centroid" <- w340
        n145 = Unbundle By Name(w340) -> ("X Centroid"=→"X centroid pos":sgl, "Y Centroid"=→"Y centroid pos":sgl)
        n146 = call "IMAQ Quantify"("error in (no error)"=w334, "Image"=w335) -> ("error out"=w333:errorcluster, "Global Report"=w332:T1)  [unwired: 1 in, 1 out]
        "Global Report" <- w332
        n147 = Unbundle By Name(w332) -> ("Maximal Value"=→"Maximal Value":sgl)
        n148 = Bundle By Name(cluster=w346, "Global Report"=w342, "Centroid"=w340, "Camera Image"=w335, "Threshold Image"=w336) -> (w345:T12)
        n149 = call <vilib>:"Add State(s) to Queue__jki_lib_state_machine.vi"("State(s) in (\"\")"=w348) -> ("States Out"=w347:string)  [unwired: 14 in]
      }
      frame #23 {
        n150 = Unbundle By Name(w356) -> ("Camera Image"=w350:T2)
        n151 = call "GaussanalysisCK.vi"("Image"=w350, "Y parameter bounds"="Y parameter bounds", "X parameter bounds"="X parameter bounds") -> ("Fit successful"=w353:bool, "Cluster"=w349:T14, "XY Graph"=→"XY Graph":cluster{i32[], "Best Gaussian Fit":dbl[]}[])  [unwired: 6 in]
        "Fit successful" <- w353
        n152 = case shown="False" w353 {
          frame #0 {
            n153 = local read "Failed Fits"() -> (w361:i32)
            n154 = Increment(x=w361) -> (x+1=w360:i32)
            n155 = local write "Failed Fits"(w360) -> ()
          }
          frame #1 {
          }
        }
        n156 = Bundle By Name(cluster=w356, "Gaussian Result"=w349) -> (w355:T12)
        n157 = call <vilib>:"Add State(s) to Queue__jki_lib_state_machine.vi"("State(s) in (\"\")"=w359) -> ("States Out"=w358:string)  [unwired: 14 in]
      }
      frame #24 {
        # "Your code here.\n(You can make a copy of, or modify, this frame)"
        n158 = call <vilib>:"Add State(s) to Queue__jki_lib_state_machine.vi"("State(s) in (\"\")"=w365) -> ("States Out"=w364:string)  [unwired: 14 in]
      }
      frame #25 {
        # "Your code here.\n(You can make a copy of, or modify, this frame)"
        n159 = call <vilib>:"Add State(s) to Queue__jki_lib_state_machine.vi"("State(s) in (\"\")"=w369) -> ("States Out"=w368:string)  [unwired: 14 in]
      }
      frame #26 {
        n160 = Unbundle By Name(w385) -> ("Framecount"=w374:u64, "IMAQdx Session"=w379:T6, "Camera Image"=w378:T2)
        n161 = Increment(x=w374) -> (x+1=w373:u64)
        n162 = call <vilib>:"IMAQdx Get Image.vi"("Buffer Number Mode (Next)"=IMAQdx_Buffer_Number_Mode."Last", "error in"=w380, "Image In"=w378, "Session In"=w379) -> ("error out"=w383:errorcluster, "Buffer Number Out"=→"Buffer Number Out":u32, "Image Out"=w370:T2, "Session Out"=w377:T6)  [unwired: 4 in]
        "Image" <- w370
        n163 = call "IMAQ ImageToArray"("error in (no error)"=w383, "Image"=w370) -> ("error out"=w375:errorcluster, "Image Pixels (I16)"=w371:i16[][])  [unwired: 2 in, 3 out]
        n164 = Add Array Elements(numeric array=w371) -> (sum=→"Waveform Chart":i16)
        n165 = Transpose 2D Array(2D array=w371) -> (transposed array=→"Intensity Graph":i16[][])
        n166 = Bundle By Name(cluster=w385, "Framecount"=w373, "IMAQdx Session"=w377, "Camera Image"=w370) -> (w384:T12)
        n167 = call <vilib>:"Add State(s) to Queue__jki_lib_state_machine.vi"("State(s) in (\"\")"=w387) -> ("States Out"=w386:string)  [unwired: 14 in]
      }
      frame #27 {
        # "Autoshutter"
        n168 = Unbundle By Name(w404) -> ("IMAQdx Session"=w393:T6, "Global Report"=w389:T1, "Camera Image"=→"Camera Image":T2)
        n169 = property class="IMAQdx"(reference=w393, error in=w392, "ActiveAttribute"="Shutter::Value") -> (reference out=w395:T6, error out=w394:errorcluster, "ValueDBL"=w396:dbl)
        "Shutter Value" <- w396
        n170 = case shown="True" "Activate Autoshutter" {
          tunnel: w389 -> [_ w418]
          tunnel: "Autoshutter Limits" -> [_ w417]
          tunnel: w394 -> [w407 w416]
          tunnel: w395 -> [w408 w415]
          tunnel: [w408 w414] -> w390
          tunnel: [w407 w413] -> w391
          tunnel: "Autoshutter Steps" -> [_ w412]
          tunnel: "ms" -> [_ w411]
          tunnel: "%" -> [_ w410]
          tunnel: w396 -> [_ w409]
          frame #0 {
          }
          frame #1 {
            n171 = call "Autoshutter.vi"("Autoshutter Steps"=w412, "%"=w410, "Autoshutter Limits"=w417, "error in"=w416, "Session in"=w415, "Global Report"=w418, "Autoshutter Value"=w409, "ms"=w411) -> ("error out"=w413:errorcluster, "Session Out"=w414:T6)  [unwired: 1 in]
          }
        }
        n172 = Bundle By Name(cluster=w404, "IMAQdx Session"=w390) -> (w403:T12)
        n173 = call <vilib>:"Add State(s) to Queue__jki_lib_state_machine.vi"("State(s) in (\"\")"=w406) -> ("States Out"=w405:string)  [unwired: 14 in]
      }
      frame #28 {
        w423 = T20 1 items=["Grayscale (U8)", "Grayscale (I16)", "Grayscale (SGL)", "Complex (CSG)", "RGB (U32)", "HSL (U32)", "RGB (U64)", "Grayscale (U16)"] ("Image Type")
        w430 = T20 1 items=["Grayscale (U8)", "Grayscale (I16)", "Grayscale (SGL)", "Complex (CSG)", "RGB (U32)", "HSL (U32)", "RGB (U64)", "Grayscale (U16)"] ("Image Type")
        n174 = call <vilib>:"IMAQdx Open Camera.vi"("Camera Control Mode"=IMAQdx_Camera_Control_Mode."Controller", "error in"=w427, "Session In"="Device") -> ("error out"=w435:errorcluster, "Session Out"=w432:T6)  [unwired: 7 in]
        n175 = call <vilib>:"IMAQdx Configure Acquisition.vi"("error in"=w435, "Number of Buffers"="Image Buffer", "Continuous?"=IMAQdx_Acquisition_Mode."Continuous", "Session In"=w432) -> ("error out"=w437:errorcluster, "Session Out"=w436:T6)  [unwired: 6 in]
        n176 = call <vilib>:"IMAQdx Start Acquisition.vi"("error in"=w437, "Session In"=w436) -> ("error out"=w428:errorcluster, "Session Out"=w426:T6)  [unwired: 8 in]
        n177 = call "IMAQ Create"("Image Name"="machiningcam", "Image Type"=w430, "error in (no error)"=w428) -> ("New Image"=w425:T2, "error out"=w421:errorcluster)  [unwired: 1 in, 1 out]
        n178 = call "IMAQ Create"("Image Name"="Treshhold", "Image Type"=w423, "error in (no error)"=w421) -> ("New Image"=w422:T2, "error out"=w420:errorcluster)  [unwired: 1 in, 1 out]
        n179 = Bundle By Name(cluster=w439, "IMAQdx Session"=w426, "Camera Image"=w425, "Threshold Image"=w422) -> (w438:T12)
        n180 = call <vilib>:"Add State(s) to Queue__jki_lib_state_machine.vi"("State(s) in (\"\")"=w441) -> ("States Out"=w440:string)  [unwired: 14 in]
      }
      frame #29 {
        n181 = Unbundle By Name(w445) -> ("IMAQdx Session"=w447:T6, "Camera Image"=w448:T2, "Threshold Image"=w442:T2)
        n182 = call "IMAQ Dispose"("Image"=w442, "error in (no error)"=w444) -> ("error out"=w443:errorcluster)  [unwired: 1 in, 3 out]
        n183 = call "IMAQ Dispose"("Image"=w448, "error in (no error)"=w443) -> ("error out"=w449:errorcluster)  [unwired: 1 in, 3 out]
        n184 = call <vilib>:"IMAQdx Stop Acquisition.vi"("error in"=w449, "Session In"=w447) -> ("error out"=w450:errorcluster)  [unwired: 8 in, 1 out]
        n185 = call <vilib>:"Simple Error Handler.vi"("error in (no error)"=w450) -> ("error out"=w446:errorcluster)  [unwired: 4 in, 4 out]
        n186 = call <vilib>:"Add State(s) to Queue__jki_lib_state_machine.vi"("State(s) in (\"\")"=w452) -> ("States Out"=w451:string)  [unwired: 14 in]
      }
    }
  }
